vi "FlatToRichcif_manager_LoaderStatus.vi"(5 "OutputClusterType":T1, 11 "InputCluster":T4) -> (3 "OutputCluster":T1)   [LabVIEW 2021, in "CIF_PluginLoader_client.lvlib"]
uses:
  CIF_PluginLoader_client.lvlib
  cif_manager_LoaderStatus_Flat.ctl
  cif_manager_LoaderInfo_Flat.ctl
  cif_manager_LoaderType.ctl
  cif_manager_LoaderStatus.ctl
  cif_manager_LoaderInfo.ctl
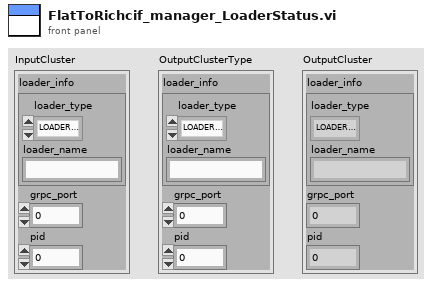
[diagram p1: front panel]
types:
  T1 = typedef "CIF_PluginLoader_client.lvlib/cif_manager_LoaderStatus.ctl" = cluster{"loader_info":T2, "grpc_port":i32, "pid":u32}
  T2 = typedef "CIF_PluginLoader_client.lvlib/cif_manager_LoaderInfo.ctl" = cluster{"loader_type":T3, "loader_name":string}
  T3 = typedef "CIF_PluginLoader_client.lvlib/cif_manager_LoaderType.ctl" = enum32{"LOADERTYPE_UNKNOWN", "LOADERTYPE_LABVIEW"}
  T4 = typedef "CIF_PluginLoader_client.lvlib/cif_manager_LoaderStatus_Flat.ctl" = cluster{"loader_info":T5, "grpc_port":i32, "pid":u32}
  T5 = typedef "CIF_PluginLoader_client.lvlib/cif_manager_LoaderInfo_Flat.ctl" = cluster{"loader_type":T3, "loader_name":string}
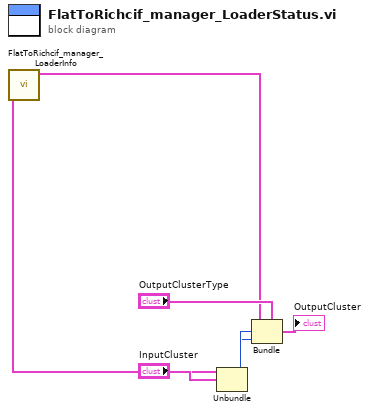
[diagram p0: block diagram]
diagram:
  n1 = Unbundle "Unbundle"("InputCluster") -> ("loader_info"=w4:T5, "grpc_port"=w2:i32, "pid"=w1:u32)
  n2 = call "FlatToRichcif_manager_LoaderInfo.vi"("InputCluster"=w4) -> ("OutputCluster"=w3:T2)  [unwired: 10 in]
  n3 = Bundle "Bundle"(cluster="OutputClusterType", "loader_info"=w3, "grpc_port"=w2, "pid"=w1) -> (→"OutputCluster":T1)
